vi "MKS670_Calib.vi"() -> ()   [LabVIEW 2019]
panel:
  in  "GPIB":enum16{"0:8", "0:7"}(ring)
  in  "dry_run":bool caption="Dry Run?"
  out "error out":errorcluster
  out "Message":string
  in  "wait":i32=30
  in  "mode":enum16{"ZERO", "NULL", "SCALE"}(ring)
  out "Status":bool
  out "Version":dbl
  out "Name":string
  # "MKS 670 Calibration"
  # "VI to do the ZERO/NULL/SCALE calibration of MKS 670.\nYou have to make the controller and/or the sensor under the proper condition for the calibration.\nIt will disable the pressure readout, and change the offset/scale of the reading.\nIf ready, you select the GPIB device name and the calibration mode, and execute this VI."
  # "0:8 = For MKS 690 / 100 Torr.\n0:7 = For MKS 615 / He3 --- Cannot be zeroed."
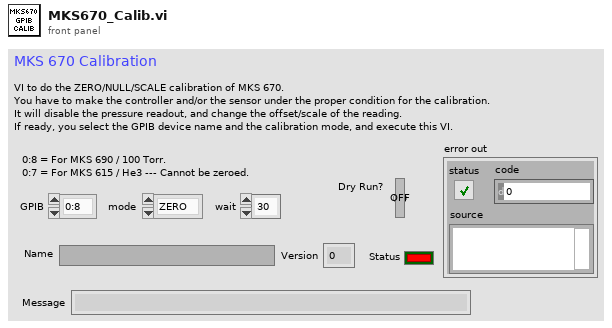
[diagram p1: front panel]
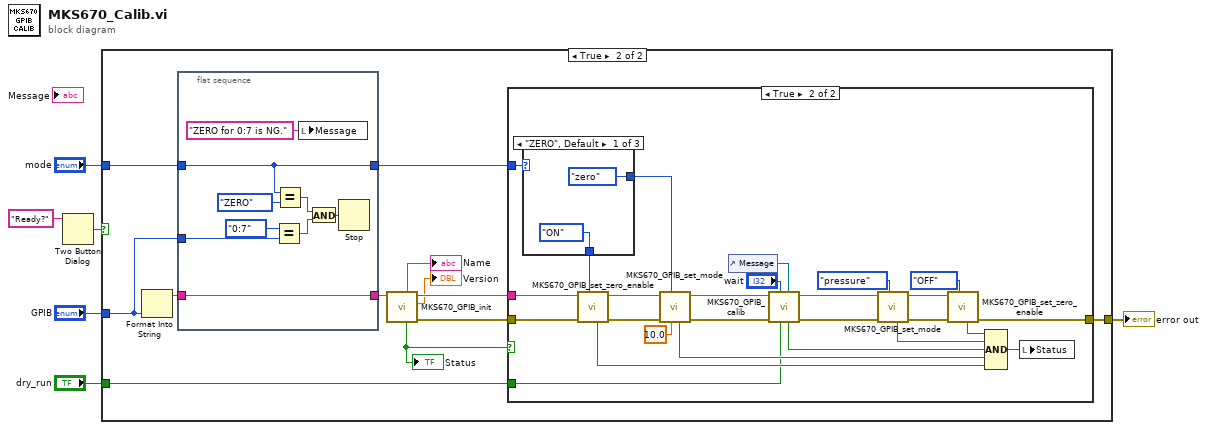
[diagram p0: block diagram]
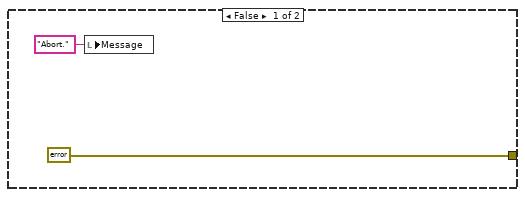
[diagram p2: hidden frame]
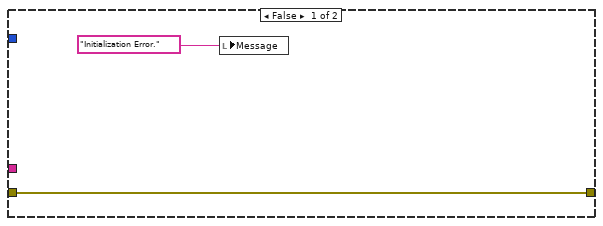
[diagram p3: hidden frame]
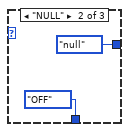
[diagram p4: hidden frame]
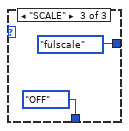
[diagram p5: hidden frame]
diagram:
  n1 = Two Button Dialog(message="Ready?") -> (T button?=w6:bool)  [unwired: 2 in]
  n2 = case shown="True" w6 {
    tunnel: "GPIB" -> [_ w12]
    tunnel: "mode" -> [_ w11]
    tunnel: "dry_run" -> [_ w10]
    tunnel: [errorcluster {"status"=FALSE, "code"=0, "source"=""} ("error out") w9] -> w1
    frame False {
      n3 = local write "Message"("Abort." ("Message")) -> ()
    }
    frame True {
      n4 = Format Into String(w12) -> (resulting string=w13:string)  [unwired: 3 in, 1 out]
      n5 = flat-sequence {
        tunnel: w11 -> [w25]
        tunnel: w13 -> [w24]
        tunnel: [w25] -> w15
        tunnel: [w24] -> w14
        tunnel: w12 -> [w22]
        frame #0 {
          n6 = Equal?(x=enum16{"0:8", "0:7"}."0:7", y=w22) -> (x = y?=w27:bool)
          n7 = Equal?(x=w25, y=enum16{"ZERO", "NULL", "SCALE"}."ZERO") -> (x = y?=w28:bool)
          n8 = local write "Message"("ZERO for 0:7 is NG." ("Message")) -> ()
          n9 = And(x=w28, y=w27) -> (x .and. y?=w26:bool)
          n10 = Stop(stop? (T)=w26) -> ()
        }
      }
      n11 = call "MKS670_GPIB_init.vi"("GPIB Address"=w14) -> ("error out"=w20:errorcluster, "Device Version"=→"Version":dbl, "GPIB out"=w19:string, "status"=w16:bool, "Device Name"=→"Name":string)  [unwired: 6 in]
      "Status" <- w16
      n12 = case shown="True" w16 {
        tunnel: w20 -> [w31 w57]
        tunnel: [w31 w48] -> w9
        tunnel: w19 -> [_ w56]
        tunnel: w10 -> [_ w36]
        tunnel: w15 -> [_ w35]
        frame False {
          n13 = local write "Message"("Initialization Error.") -> ()
        }
        frame True {
          n14 = case shown="\"ZERO\", Default" w35 {
            tunnel: [enum16{"pressure", "zero", "null", "fulscale"}."zero" ("mode") enum16{"pressure", "zero", "null", "fulscale"}."null" ("mode") enum16{"pressure", "zero", "null", "fulscale"}."fulscale" ("mode")] -> w34
            tunnel: [enum16{"ON", "OFF"}."ON" ("mode") enum16{"ON", "OFF"}."OFF" ("mode") enum16{"ON", "OFF"}."OFF" ("mode")] -> w33
            frame "ZERO", Default {
            }
            frame "NULL" {
            }
            frame "SCALE" {
            }
          }
          n15 = call "MKS670_GPIB_set_zero_enable.vi"("mode"=w33, "error in"=w57, "GPIB in"=w56) -> ("error out"=w54:errorcluster, "GPIB out"=w53:string, "status"=w37:bool)  [unwired: 6 in]
          n16 = call "MKS670_GPIB_set_mode.vi"("wait"=10.0, "mode"=w34, "error in"=w54, "GPIB in"=w53) -> ("error out"=w52:errorcluster, "GPIB out"=w51:string, "status"=w38:bool)  [unwired: 5 in]
          n17 = control-ref of="Message"() -> (w43:refnum<vi>)
          n18 = call "MKS670_GPIB_calib.vi"("ref_msg"=w43, "dry_run"=w36, "wait"="wait", "error in"=w52, "GPIB in"=w51) -> ("error out"=w50:errorcluster, "GPIB out"=w47:string, "status"=w39:bool)  [unwired: 4 in]
          n19 = call "MKS670_GPIB_set_mode.vi"("mode"=enum16{"pressure", "zero", "null", "fulscale"}."pressure", "error in"=w50, "GPIB in"=w47) -> ("error out"=w49:errorcluster, "GPIB out"=w46:string, "status"=w40:bool)  [unwired: 6 in]
          n20 = call "MKS670_GPIB_set_zero_enable.vi"("mode"=enum16{"ON", "OFF"}."OFF", "error in"=w49, "GPIB in"=w46) -> ("error out"=w48:errorcluster, "status"=w41:bool)  [unwired: 6 in, 1 out]
          n21 = Compound Arithmetic op=AND(w41, w40, w39, w38, w37) -> (w42:bool)
          n22 = local write "Status"(w42) -> ()
        }
      }
    }
  }
  "error out" <- w1
